vi "Untitled 3.vi"() -> ()   [LabVIEW 2021]
uses:
  <vilib>/Utility/file.llb/Read Delimited Spreadsheet (DBL).vi
  <vilib>/Analysis/NI_AALBase.lvlib
  <vilib>/gmath/NI_Gmath.lvlib
  <vilib>/Utility/file.llb/Write Delimited Spreadsheet (DBL).vi
panel:
  out "Last FAA Resistance":dbl format="%0.2f"
  out "Last GGG Resistance":dbl format="%0.2f"
  out "Temperature Plot":cluster{timestamp[], dbl[]}[](graph)
  in  "Moving Median Size":i32=25
  in  "FAA Calibration FIle":path
  in  "GGG Calibration File":path
  in  "VISA RESOURCE":refnum<visa-resource-name>="COM5"
  in  "EXCITATION":u8(ring)=4 items=["0", "3 uV", "10 uV", "30 uV", "100 uV", "300 uV", "1 mV", "3 mV"]
  in  "Temperature Log File Path":path
  in  "?":bool
  in  "Time Between GGG Measurements":dbl(ring)=300.0 items=["30 s"=30.0, "1 m"=60.0, "2 m"=120.0, "5 m"=300.0, "10 m"=600.0, "20 m"=1200.0, "30 m"=1800.0, "1 h"=3600.0, "2 h"=7200.0]
  in  "Override":bool
  in  "Override":T1
  in  "Number of GGG Samples":i32=20
  in  "?":bool
  out "Last GGG Temp":dbl
  out "Last FAA Temp":dbl
  out "Raw Resistance":dbl
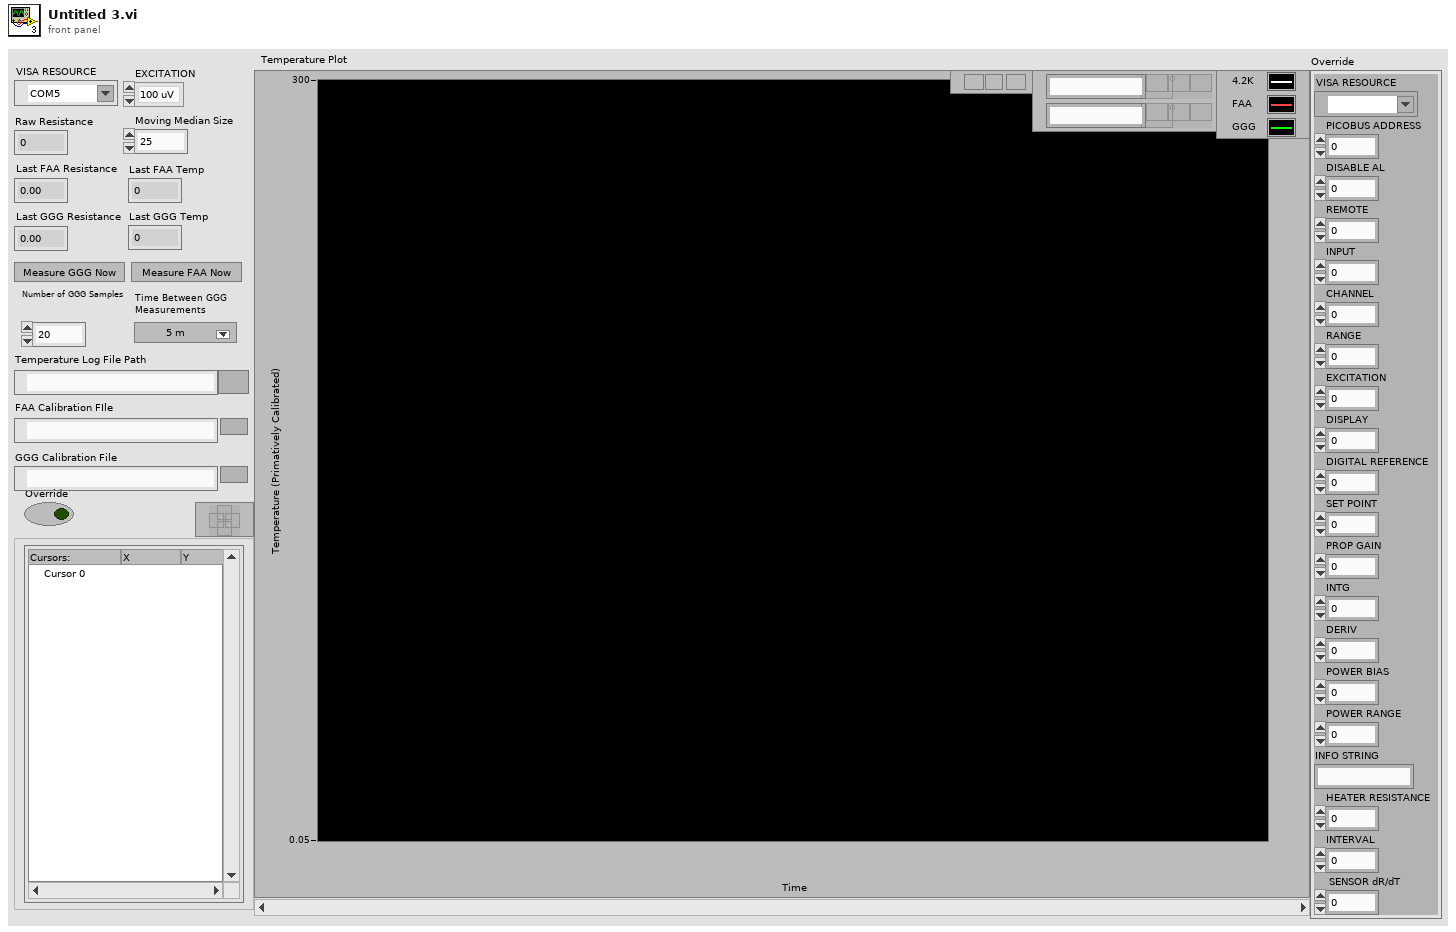
[diagram p1: front panel]
types:
  T1 = cluster{"VISA RESOURCE":refnum<visa-resource-name>, "PICOBUS ADDRESS":u8, "DISABLE AL":u8, "REMOTE":u8, "INPUT":u8, "CHANNEL":u8, "RANGE":u8, "EXCITATION":u8, "DISPLAY":u8, "DIGITAL REFERENCE":u16, "SET POINT":dbl, "PROP GAIN":u8, "INTG":u8, "DERIV":u8, "POWER BIAS":u8, "POWER RANGE":u8, "INFO STRING":string, "HEATER RESISTANCE":dbl, "INTERVAL":u8, " SENSOR dR/dT":u8}
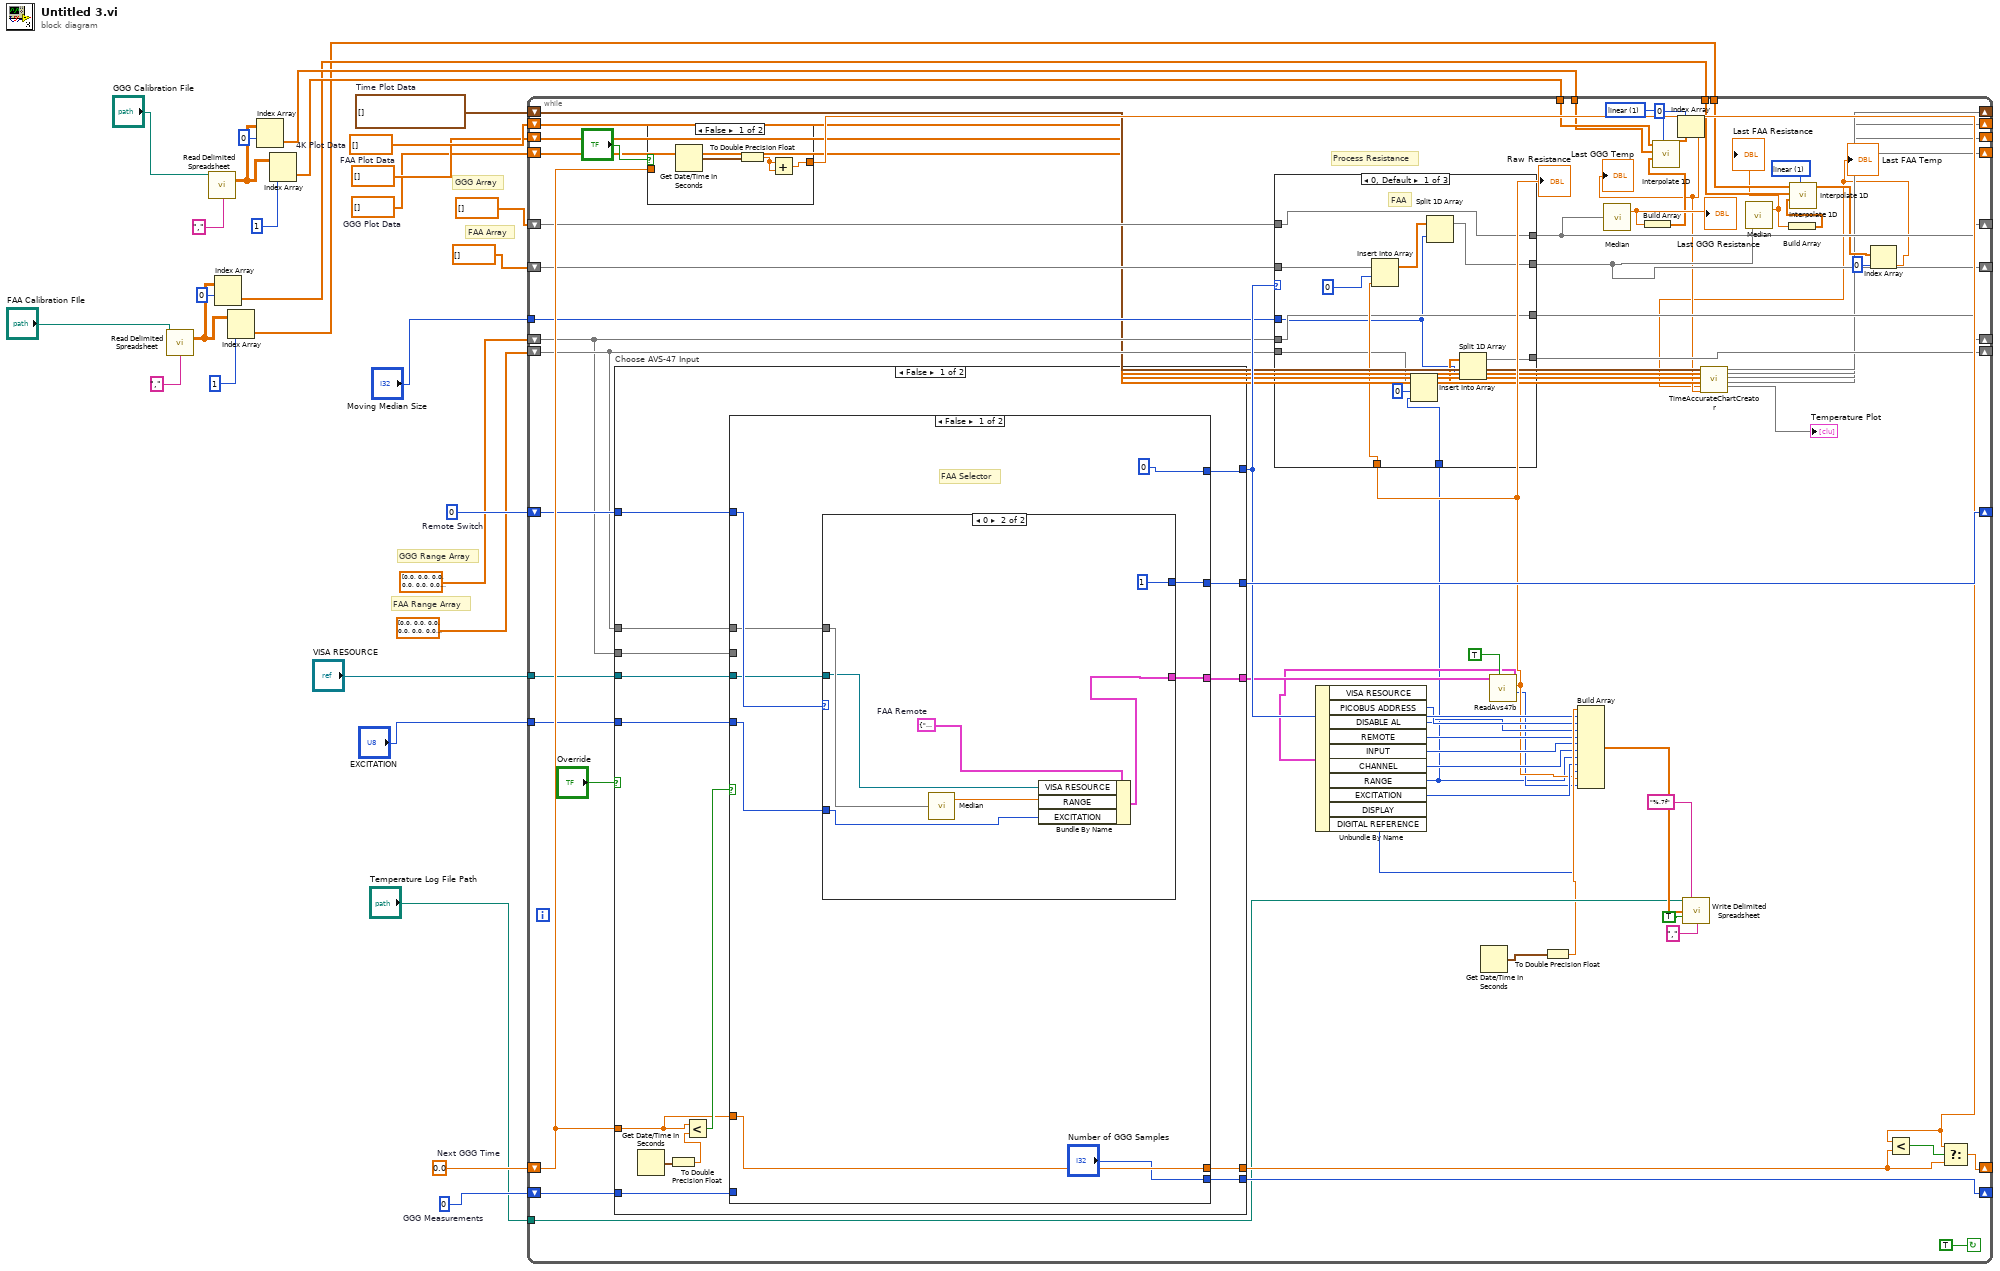
[diagram p0: block diagram]
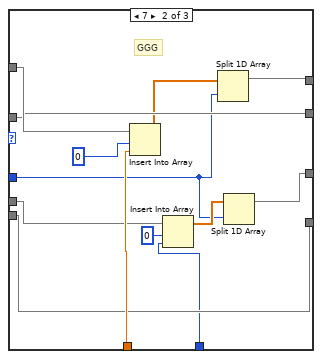
[diagram p2: hidden frame]
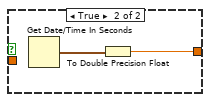
[diagram p4: hidden frame]
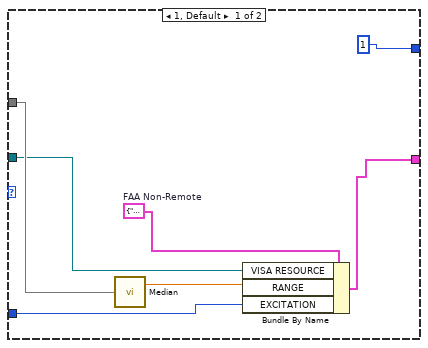
[diagram p5: hidden frame]
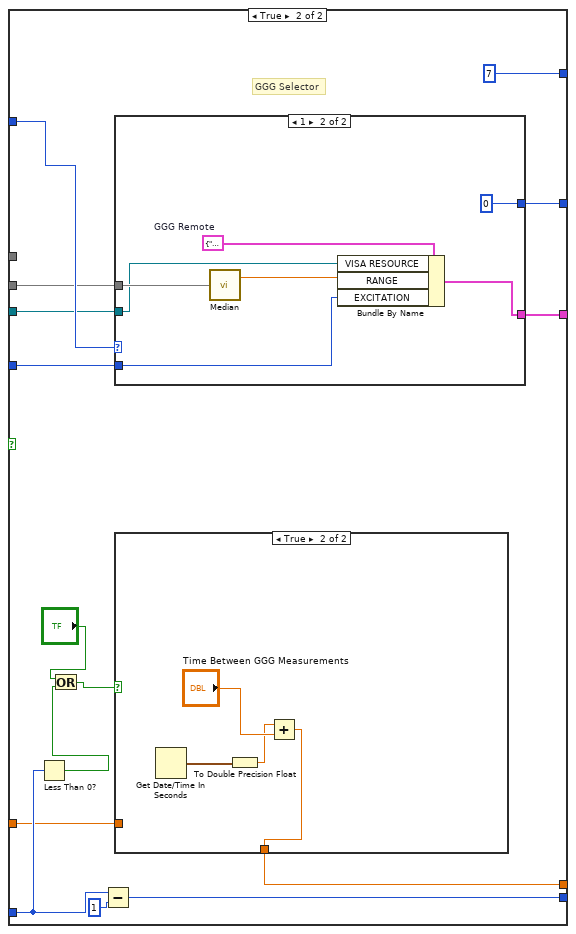
[diagram p6: hidden frame]
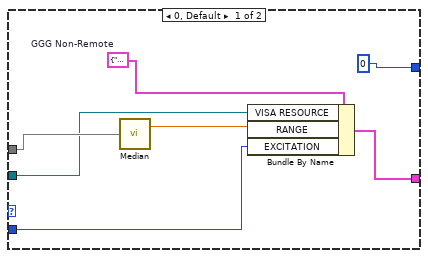
[diagram p8: hidden frame]
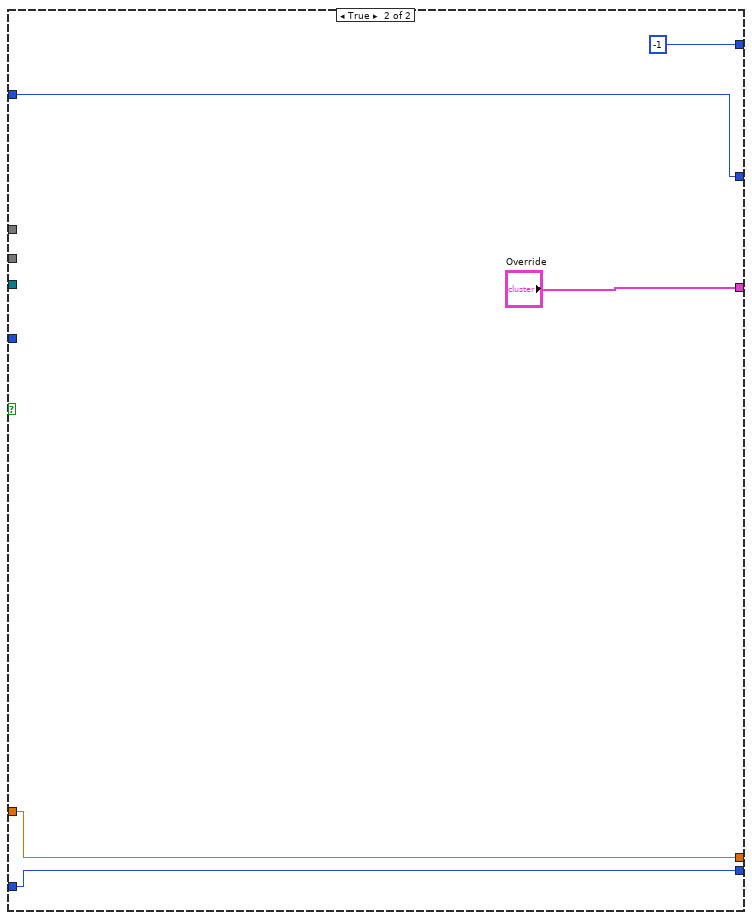
[diagram p9: hidden frame]
diagram:
  w1 = dbl[] []  # GGG Plot Data
  w2 = dbl[] []  # FAA Plot Data
  w3 = dbl[] []  # 4K Plot Data
  w4 = timestamp[] []  # Time Plot Data
  w27 = 0  # GGG Measurements
  w28 = 0  # Remote Switch
  w29 = 0.0  # Next GGG Time
  # "FAA Range Array"
  # "GGG Range Array"
  # "FAA Array"
  # "GGG Array"
  n1 = call-poly <vilib>:"Read Delimited Spreadsheet.vi"("file path (dialog if empty)"="FAA Calibration FIle", "delimiter (\\t)"="," ("delimiter (\\t)")) -> ("all rows"=w18:dbl[][])  [unwired: 8 in, 5 out]
  n2 = call-poly <vilib>:"Read Delimited Spreadsheet.vi"("file path (dialog if empty)"="GGG Calibration File", "delimiter (\\t)"="," ("delimiter (\\t)")) -> ("all rows"=w22:dbl[][])  [unwired: 8 in, 5 out]
  n3 = Index Array(array=w18, index (row)=0) -> (element=w14:dbl[])  [unwired: 1 in]
  n4 = Index Array(array=w18, index (row)=1) -> (element=w13:dbl[])  [unwired: 1 in]
  n5 = Index Array(array=w22, index (row)=0) -> (element=w16:dbl[])  [unwired: 1 in]
  n6 = Index Array(array=w22, index (row)=1) -> (element=w15:dbl[])  [unwired: 1 in]
  n7 = while {
    shift-right: [w91] -> _
    shift-left: w29 -> [w96]
    shift-right: [w94] -> _
    shift-left: w28 -> [w95]
    shift-right: [w92] -> _
    shift-left: w27 -> [w93]
    shift-right: [w83] -> _
    shift-left: sgl[] [] ("array") -> [w85]
    shift-right: [w82] -> _
    shift-left: sgl[] [] ("array") -> [w84]
    tunnel: w16 -> [w54]
    tunnel: w15 -> [w55]
    tunnel: w14 -> [w61]
    tunnel: w13 -> [w62]
    tunnel: "Temperature Log File Path" -> [w76]
    tunnel: "EXCITATION" -> [w48]
    shift-right: [w47] -> _
    shift-left: sgl[] [0.0, 0.0, 0.0, 0.0, 0.0, 0.0, 0.0, 0.0, 0.0, 0.0, 3.0] ("array") -> [w42]
    shift-right: [w46] -> _
    shift-left: sgl[] [0.0, 0.0, 0.0, 0.0, 0.0, 0.0, 0.0, 0.0, 0.0, 0.0, 3.0] ("array") -> [w43]
    tunnel: "VISA RESOURCE" -> [w44]
    tunnel: "Moving Median Size" -> [w41]
    shift-right: [w39] -> _
    shift-left: w4 -> [w40]
    shift-right: [w33] -> _
    shift-left: w3 -> [w38]
    shift-right: [w32] -> _
    shift-left: w2 -> [w37]
    shift-right: [w31] -> _
    shift-left: w1 -> [w36]
    stop <- TRUE continue-if-true
    w51 = 1 items=["nearest", "linear", "spline", "cubic Hermite", "Lagrange"] ("method")
    w56 = 1 items=["nearest", "linear", "spline", "cubic Hermite", "Lagrange"] ("method")
    # "Process Resistance"
    n8 = case "Choose AVS-47 Input" shown="False" "Override" {
      tunnel: w96 -> [w139 w207]
      tunnel: w95 -> [w145 w209]
      tunnel: [w144 "Override"] -> w73
      tunnel: [w143 w209] -> w94
      tunnel: w93 -> [w142 w206]
      tunnel: [w141 w206] -> w92
      tunnel: [w140 w207] -> w89
      tunnel: [w138 -1] -> w74
      tunnel: w48 -> [w137 _]
      tunnel: w42 -> [w136 _]
      tunnel: w43 -> [w135 _]
      tunnel: w44 -> [w134 _]
      frame False {
        n9 = Get Date/Time In Seconds() -> (seconds since 1Jan1904=w148:timestamp)
        n10 = To Double Precision Float(number=w148) -> (double precision float=w147:dbl)
        n11 = Less?(x=w139, y=w147) -> (x < y?=w146:bool)
        n12 = case shown="False" w146 {
          tunnel: w145 -> [w157 w186]
          tunnel: [w155 w185] -> w144
          tunnel: [w156 w184] -> w143
          tunnel: w142 -> [_ w181]
          tunnel: ["Number of GGG Samples" w182] -> w141
          tunnel: [w154 w180] -> w140
          tunnel: w139 -> [w154 w179]
          tunnel: [0 7] -> w138
          tunnel: w137 -> [w151 w174]
          tunnel: w136 -> [_ w173]
          tunnel: w135 -> [w150 _]
          tunnel: w134 -> [w149 w172]
          frame False {
            # "FAA Selector"
            n13 = case shown="0" w157 {
              tunnel: [w161 w166] -> w155
              tunnel: [1 1] -> w156
              tunnel: w151 -> [w160 w167]
              tunnel: w150 -> [w159 w168]
              tunnel: w149 -> [w158 w165]
              frame 1, Default {
                w162 = T1 {"VISA RESOURCE"="COM5", "PICOBUS ADDRESS"=1, "DISABLE AL"=0, "REMOTE"=0, "INPUT"=1, "CHANNEL"=0, "RANGE"=5, "EXCITATION"=4, "DISPLAY"=0, "DIGITAL REFERENCE"=0, "SET POINT"=0.0, "PROP GAIN"=0, "INTG"=0, "DERIV"=0, "POWER BIAS"=0, "POWER RANGE"=0, "INFO STRING"="", "HEATER RESISTANCE"=0.0, "INTERVAL"=0, " SENSOR dR/dT"=0}  # FAA Non-Remote
                n14 = call <vilib>:"Median.vi"("X"=w159) -> ("median"=w163:dbl)  [unwired: 1 out]
                n15 = Bundle By Name(cluster=w162, "VISA RESOURCE"=w158, "RANGE"=w163, "EXCITATION"=w160) -> (w161:T1)
              }
              frame 0 {
                w169 = T1 {"VISA RESOURCE"="COM5", "PICOBUS ADDRESS"=1, "DISABLE AL"=0, "REMOTE"=1, "INPUT"=1, "CHANNEL"=0, "RANGE"=5, "EXCITATION"=4, "DISPLAY"=0, "DIGITAL REFERENCE"=0, "SET POINT"=0.0, "PROP GAIN"=0, "INTG"=0, "DERIV"=0, "POWER BIAS"=0, "POWER RANGE"=0, "INFO STRING"="", "HEATER RESISTANCE"=0.0, "INTERVAL"=0, " SENSOR dR/dT"=0}  # FAA Remote
                n16 = call <vilib>:"Median.vi"("X"=w168) -> ("median"=w170:dbl)  [unwired: 1 out]
                n17 = Bundle By Name(cluster=w169, "VISA RESOURCE"=w165, "RANGE"=w170, "EXCITATION"=w167) -> (w166:T1)
              }
            }
          }
          frame True {
            # "GGG Selector"
            n18 = Less Than 0?(x=w181) -> (x < 0?=w178:bool)
            n19 = Or(x="?", y=w178) -> (x .or. y?=w176:bool)
            n20 = Subtract(x=w181, y=1) -> (x-y=w182:i32)
            n21 = case shown="1" w186 {
              tunnel: [w193 w202] -> w185
              tunnel: [0 0] -> w184
              tunnel: w174 -> [w194 w204]
              tunnel: w173 -> [w195 w201]
              tunnel: w172 -> [w192 w199]
              frame 0, Default {
                w196 = T1 {"VISA RESOURCE"="COM5", "PICOBUS ADDRESS"=1, "DISABLE AL"=0, "REMOTE"=0, "INPUT"=1, "CHANNEL"=7, "RANGE"=4, "EXCITATION"=4, "DISPLAY"=0, "DIGITAL REFERENCE"=0, "SET POINT"=0.0, "PROP GAIN"=0, "INTG"=0, "DERIV"=0, "POWER BIAS"=0, "POWER RANGE"=0, "INFO STRING"="", "HEATER RESISTANCE"=0.0, "INTERVAL"=0, " SENSOR dR/dT"=0}  # GGG Non-Remote
                n22 = call <vilib>:"Median.vi"("X"=w195) -> ("median"=w197:dbl)  [unwired: 1 out]
                n23 = Bundle By Name(cluster=w196, "VISA RESOURCE"=w192, "RANGE"=w197, "EXCITATION"=w194) -> (w193:T1)
              }
              frame 1 {
                w203 = T1 {"VISA RESOURCE"="COM5", "PICOBUS ADDRESS"=1, "DISABLE AL"=0, "REMOTE"=1, "INPUT"=1, "CHANNEL"=7, "RANGE"=4, "EXCITATION"=4, "DISPLAY"=0, "DIGITAL REFERENCE"=0, "SET POINT"=0.0, "PROP GAIN"=0, "INTG"=0, "DERIV"=0, "POWER BIAS"=0, "POWER RANGE"=0, "INFO STRING"="", "HEATER RESISTANCE"=0.0, "INTERVAL"=0, " SENSOR dR/dT"=0}  # GGG Remote
                n24 = call <vilib>:"Median.vi"("X"=w201) -> ("median"=w200:dbl)  [unwired: 1 out]
                n25 = Bundle By Name(cluster=w203, "VISA RESOURCE"=w199, "RANGE"=w200, "EXCITATION"=w204) -> (w202:T1)
              }
            }
            n26 = case shown="True" w176 {
              tunnel: [w187 w188] -> w180
              tunnel: w179 -> [w187 _]
              frame False {
              }
              frame True {
                n27 = Get Date/Time In Seconds() -> (seconds since 1Jan1904=w191:timestamp)
                n28 = To Double Precision Float(number=w191) -> (double precision float=w189:dbl)
                n29 = Add(x=w189, y="Time Between GGG Measurements") -> (x+y=w188:dbl)
              }
            }
          }
        }
      }
      frame True {
      }
    }
    n30 = case shown="False" "?" {
      tunnel: [w130 w132] -> w90
      tunnel: w96 -> [_ _]
      frame False {
        n31 = Get Date/Time In Seconds() -> (seconds since 1Jan1904=w131:timestamp)
        n32 = To Double Precision Float(number=w131) -> (double precision float=w129:dbl)
        n33 = Add(x=w129, y=w129) -> (x+y=w130:dbl)
      }
      frame True {
        n34 = Get Date/Time In Seconds() -> (seconds since 1Jan1904=w133:timestamp)
        n35 = To Double Precision Float(number=w133) -> (double precision float=w132:dbl)
      }
    }
    n36 = Get Date/Time In Seconds() -> (seconds since 1Jan1904=w81:timestamp)
    n37 = call "ReadAvs47b.vi"("SYNCHRONISE TO ADC"=TRUE, "CONFIGURATION CLUSTER"=w73) -> ("ADC"=w64:i32, "RESISTANCE (OHMS)"=w65:sgl, "MODIFIED CONFIGURATION CLUSTER"=w63:T1)  [unwired: 4 in, 3 out]
    "Raw Resistance" <- w65
    n38 = Unbundle By Name(w63) -> ("PICOBUS ADDRESS"=w72:u8, "DISABLE AL"=w71:u8, "REMOTE"=w70:u8, "INPUT"=w69:u8, "CHANNEL"=w68:u8, "RANGE"=w45:u8, "EXCITATION"=w67:u8, "DISPLAY"=w66:u8)  [unwired: 2 out]
    n39 = case shown="0, Default" w74 {
      tunnel: w65 -> [w108 w124 _]
      tunnel: w85 -> [w109 w122 w128]
      tunnel: w84 -> [w110 w121 w127]
      tunnel: [w109 w116 w128] -> w83
      tunnel: [w103 w121 w127] -> w82
      tunnel: w42 -> [w107 w119 w126]
      tunnel: w43 -> [w104 w120 w125]
      tunnel: [w107 w113 w126] -> w47
      tunnel: [w99 w120 w125] -> w46
      tunnel: w45 -> [w105 w117 _]
      tunnel: w41 -> [w100 w112 _]
      frame 0, Default {
        # "FAA"
        n40 = Insert Into Array(array=w110, index=0, new element=w108) -> (w102:sgl[])
        n41 = Insert Into Array(array=w104, index=0, new element=w105) -> (w101:sgl[])
        n42 = Split 1D Array(array=w102, index=w100) -> (first subarray=w103:sgl[])  [unwired: 1 out]
        n43 = Split 1D Array(array=w101, index=w100) -> (first subarray=w99:sgl[])  [unwired: 1 out]
      }
      frame 7 {
        # "GGG"
        n44 = Insert Into Array(array=w122, index=0, new element=w124) -> (w115:sgl[])
        n45 = Insert Into Array(array=w119, index=0, new element=w117) -> (w114:sgl[])
        n46 = Split 1D Array(array=w115, index=w112) -> (first subarray=w116:sgl[])  [unwired: 1 out]
        n47 = Split 1D Array(array=w114, index=w112) -> (first subarray=w113:sgl[])  [unwired: 1 out]
      }
      frame -1 {
      }
    }
    n48 = To Double Precision Float(number=w81) -> (double precision float=w75:dbl)
    n49 = Build Array(w75, w74, w72, w71, w70, w69, w68, w45, w67, w66, w65, w64) -> (w80:dbl[])
    n50 = call <vilib>:"Median.vi"("X"=w83) -> ("median"=w53:dbl)  [unwired: 1 out]
    "Last GGG Resistance" <- w53
    n51 = Build Array(w53) -> (w52:dbl[])
    n52 = call <vilib>:"Interpolate 1D.vi"("method"=w51, "xi"=w52, "X"=w54, "Y"=w55) -> ("yi"=w50:dbl[])  [unwired: 5 in, 2 out]
    n53 = Index Array(array=w50, index=0) -> (element=w35:dbl)
    "Last GGG Temp" <- w35
    n54 = call-poly <vilib>:"Write Delimited Spreadsheet.vi"("file path (dialog if empty)"=w76, "format (%.3f)"="%.7f", "1D data"=w80, "append to file? (new file:F)"=TRUE, "delimiter (\\t)"="," ("delimiter (\\t)")) -> ()  [unwired: 9 in, 2 out]
    n55 = call <vilib>:"Median.vi"("X"=w82) -> ("median"=w60:dbl)  [unwired: 1 out]
    "Last FAA Resistance" <- w60
    n56 = Build Array(w60) -> (w59:dbl[])
    n57 = call <vilib>:"Interpolate 1D.vi"() -> ()  [unwired: 9 in, 3 out]
    n58 = call <vilib>:"Interpolate 1D.vi"("method"=w56, "xi"=w59, "X"=w61, "Y"=w62) -> ("yi"=w57:dbl[])  [unwired: 5 in, 2 out]
    n59 = Index Array(array=w57, index=0) -> (element=w34:dbl)
    "Last FAA Temp" <- w34
    n60 = call "TimeAccurateChartCreator.vi"(0:w40, 1:w38, 2:w37, 3:w36, 4:w34, 5:w35) -> (14:w39, 15:w33, 16:w32, 17:w31, 18:→"Temperature Plot")  [unwired: 9 in]
    n61 = Less?(x=w90, y=w89) -> (x < y?=w88:bool)
    n62 = Select(t=w90, s=w88, f=w89) -> (s? t:f=w91:dbl)
  }
